vi "no_info.vi"() -> ()   [LabVIEW 2019]
panel:
  out "concatenated string":string
  in  "Numeric":dbl
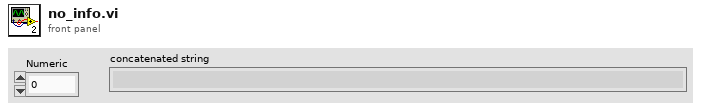
[diagram p1: front panel]
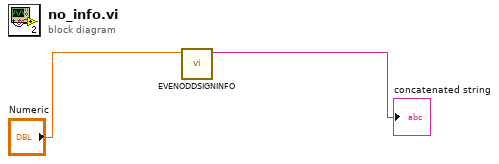
[diagram p0: block diagram]
diagram:
  n1 = call "EVENODDSIGNINFO.vi"("Numeric"="Numeric") -> ("concatenated string"=→"concatenated string":string)  [unwired: 10 in]
